vi "Supports Block Diagram.vi"(8 "error in (no error)":errorcluster, 11 "vi in":refnum<vi>) -> (0 "error out":errorcluster, 2 "has block diagram":bool, 3 "vi out":refnum<vi>)   [LabVIEW 2024]
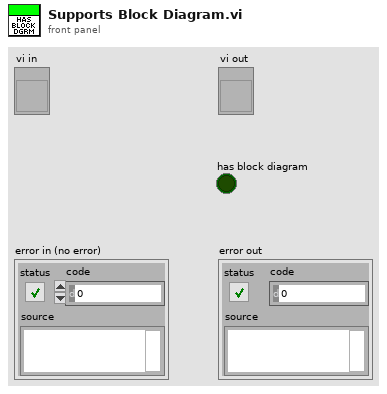
[diagram p1: front panel]
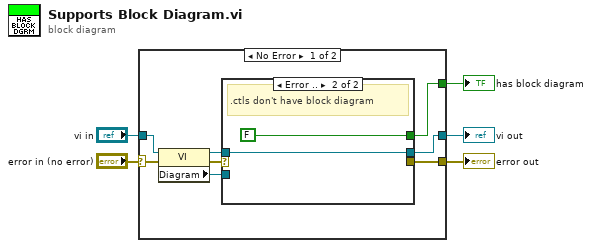
[diagram p0: block diagram]
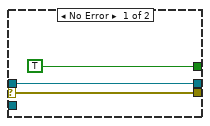
[diagram p2: hidden frame]
diagram:
  n1 = case shown="No Error" "error in (no error)" {
    selector: "error in (no error)" -> [w12 w20]
    tunnel: [w8 w19] -> w5
    tunnel: [w7 w20] -> w4
    tunnel: "vi in" -> [w13 w19]
    tunnel: [w6 _] -> w1
    frame No Error {
      n2 = property class="VI"(reference=w13, error in=w12) -> (reference out=w11:refnum<vi>, error out=w10:errorcluster, "Diagram"=w9:refnum<vi>)
      n3 = case shown="Error .." w10 {
        selector: w10 -> [w15 _]
        tunnel: w11 -> [w16 w18]
        tunnel: w9 -> [_ _]
        tunnel: [w16 w18] -> w8
        tunnel: [w15 _] -> w7
        tunnel: [TRUE FALSE] -> w6
        frame No Error {
        }
        frame Error {
          # ".ctls don't have block diagram"
        }
      }
    }
    frame Error {
    }
  }
  "vi out" <- w5
  "error out" <- w4
  "has block diagram" <- w1
